vi "stop.vi"(8 "error in (no error)":errorcluster, 10 "stop":bool, 11 "DIO64Output in":refnum<class "DIO64Output.lvclass">) -> (0 "error out":errorcluster, 2 "Stopped?":bool, 3 "DIO64Output out":refnum<class "DIO64Output.lvclass">)   [LabVIEW 2009, in "Hardware.lvlib" / "Channels.lvlib" / "DIO64Output.lvclass"]
uses:
  DIO64Output.lvclass
  DIO64Output.lvclass/DIO64Output.ctl
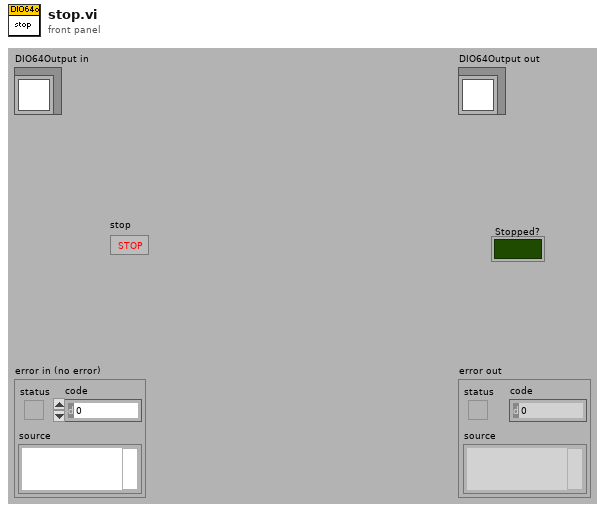
[diagram p1: front panel]
types:
  T1 = cluster{"Master Clock source":string, "Master Clock rate":dbl, "Start trigger line":string, "Scan rate":dbl, "Stop trigger line":string, "Sample Number":dbl}
  T2 = typedef "DIO64 Out Status.ctl" = cluster{"pktsize":u16, "portCount":u16, "writePtr":u16, "readPtr":u16, "time0":u16, "time1":u16, "fifoSize":u32, "fifo0":u16, "ticks":u32, "flags":u16, "clkControl":u16, "startControl":u16, "stopControl":u16, "AIControl":u32, "AICurrent":u16, "startTime0":u16, "startTime1":u16, "stopTime0":u16, "stopTime1":u16, "cur trans":u32, "cur reps":u32}
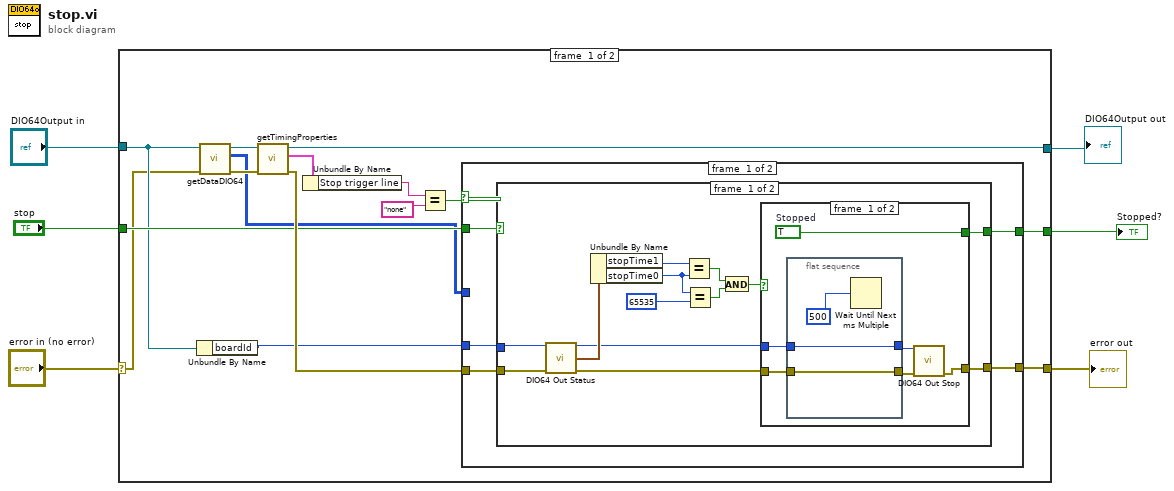
[diagram p0: block diagram]
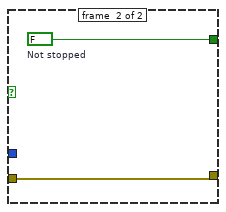
[diagram p2: hidden frame]
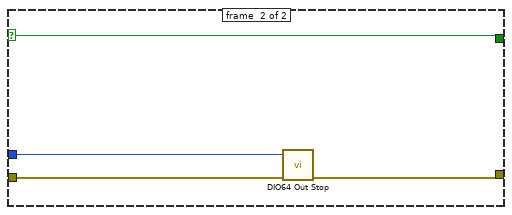
[diagram p3: hidden frame]
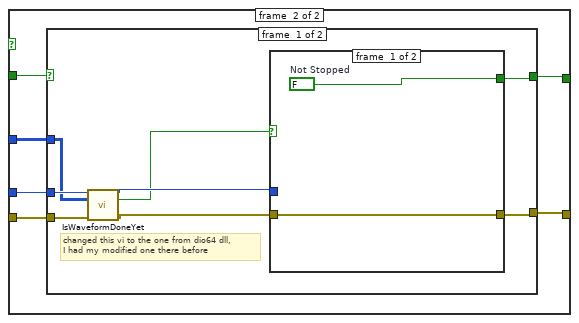
[diagram p4: hidden frame]
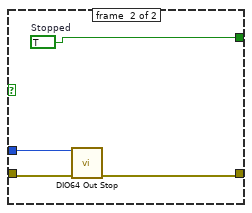
[diagram p5: hidden frame]
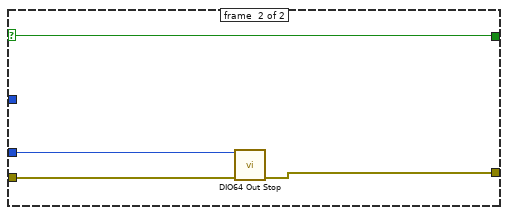
[diagram p6: hidden frame]
diagram:
  n1 = case shown="No Error" "error in (no error)" {
    selector: "error in (no error)" -> [w7 w81]
    tunnel: [w21 w81] -> w3
    tunnel: "DIO64Output in" -> [w9 w80]
    tunnel: [w19 w80] -> w4
    tunnel: "stop" -> [w14 w79]
    tunnel: [w13 w79] -> w1
    frame #0 {
      n2 = Unbundle By Name(w9) -> ("boardId"=w8:i32)
      n3 = call "getDataDIO64.vi"("error in (no error)"=w7, "DIO64Output.lvclass in"=w9) -> ("error out"=w12:errorcluster, "data"=w10:u16[][], "DIO64Output.lvclass out"=w11:refnum<class "DIO64Output.lvclass">)  [unwired: 7 in]
      n4 = call-dynamic "getTimingProperties.vi"("error in (no error)"=w12, "DigitalOutput.lvclass in"=w11) -> ("error out"=w20:errorcluster, "Timing"=w18:T1, "DigitalOutput.lvclass out"=w19:refnum<class "DIO64Output.lvclass">)  [unwired: 7 in]
      n5 = Unbundle By Name(w18) -> ("Stop trigger line"=w16:string)
      n6 = Equal?(x=w16, y="none") -> (x = y?=w15:bool)
      n7 = case shown="True" w15 {
        tunnel: [w24 w58] -> w21
        tunnel: w8 -> [w26 w60]
        tunnel: w20 -> [w25 w59]
        tunnel: w14 -> [w23 w56]
        tunnel: [w22 w57] -> w13
        tunnel: w10 -> [_ w55]
        frame #0 {
          n8 = case shown="False" w23 {
            selector: w23 -> [_ w54]
            tunnel: w26 -> [w39 w52]
            tunnel: w25 -> [w38 w53]
            tunnel: [w27 w51] -> w24
            tunnel: [w30 w54] -> w22
            frame #0 {
              n9 = call <userlib>:"DIO64 Out Status.vi"("board in"=w39, "error in (no error)"=w38) -> ("board out"=w29:u16, "Out Status"=w37:T2, "error out"=w28:errorcluster)  [unwired: 10 in, 1 out]
              n10 = Unbundle By Name(w37) -> ("stopTime1"=w36:u16, "stopTime0"=w35:u16)
              n11 = Equal?(x=w36, y=w35) -> (x = y?=w32:bool)
              n12 = Equal?(x=w35, y=65535) -> (x = y?=w31:bool)
              n13 = And(x=w32, y=w31) -> (x .and. y?=w33:bool)
              n14 = case shown="False" w33 {
                tunnel: [w45 w50] -> w30
                tunnel: w29 -> [w44 _]
                tunnel: w28 -> [w43 w49]
                tunnel: [w41 w49] -> w27
                frame #0 {
                  w45 = TRUE  # Stopped
                  n15 = flat-sequence {
                    tunnel: w44 -> [w47]
                    tunnel: [w47] -> w40
                    tunnel: w43 -> [w46]
                    tunnel: [w46] -> w42
                    frame #0 {
                      n16 = Wait Until Next ms Multiple(millisecond multiple=500) -> ()  [unwired: 1 out]
                    }
                  }
                  n17 = call <userlib>:"DIO64 Out Stop.vi"("board in"=w40, "error in (no error)"=w42) -> ("error out"=w41:errorcluster)  [unwired: 12 in, 1 out]
                }
                frame #1 {
                  w50 = FALSE  # Not stopped
                }
              }
            }
            frame #1 {
              n18 = call <userlib>:"DIO64 Out Stop.vi"("board in"=w52, "error in (no error)"=w53) -> ("error out"=w51:errorcluster)  [unwired: 12 in, 1 out]
            }
          }
        }
        frame #1 {
          n19 = case shown="False" w56 {
            selector: w56 -> [_ w78]
            tunnel: w60 -> [w64 w77]
            tunnel: w59 -> [w65 w76]
            tunnel: [w67 w75] -> w58
            tunnel: [w68 w78] -> w57
            tunnel: w55 -> [w61 _]
            frame #0 {
              # "changed this vi to the one from dio64 dll,\nI had my modified one there before"
              n20 = call <userlib>:"IsWaveformDoneYet.vi"("board in"=w64, "data"=w61, "error in (no error)"=w65) -> ("board out"=w63:u16, "waveform done?"=w62:bool, "error out"=w66:errorcluster)  [unwired: 10 in]
              n21 = case shown="True" w62 {
                tunnel: [w70 w74] -> w68
                tunnel: [w69 w71] -> w67
                tunnel: w66 -> [w69 w73]
                tunnel: w63 -> [_ w72]
                frame #0 {
                  w70 = FALSE  # Not Stopped
                }
                frame #1 {
                  w74 = TRUE  # Stopped
                  n22 = call <userlib>:"DIO64 Out Stop.vi"("board in"=w72, "error in (no error)"=w73) -> ("error out"=w71:errorcluster)  [unwired: 12 in, 1 out]
                }
              }
            }
            frame #1 {
              n23 = call <userlib>:"DIO64 Out Stop.vi"("board in"=w77, "error in (no error)"=w76) -> ("error out"=w75:errorcluster)  [unwired: 12 in, 1 out]
            }
          }
        }
      }
    }
    frame #1 {
    }
  }
  "error out" <- w3
  "DIO64Output out" <- w4
  "Stopped?" <- w1
